vi "Day 14-Add to Pair Count.vi"(8 "Count":u64, 9 "Pair 2":u8[](array[numeric]), 10 "Pair 1":u8[](array[numeric]), 11 "Count in":map{u8[], u64}(c390)) -> (3 "Count out":map{u8[], u64}(c390))   [LabVIEW 2021]
uses:
  <vilib>/Utility/miscctls.llb/LVMapReplaceAction.ctl
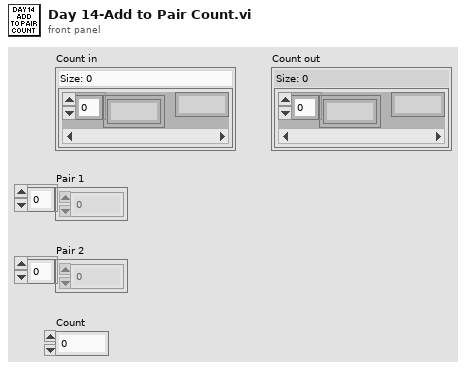
[diagram p1: front panel]
types:
  T1 = typedef "LVMapReplaceAction.ctl" = enum32{"Modify Entry only if found", "Add or Modify Entry", "Delete Entry"}
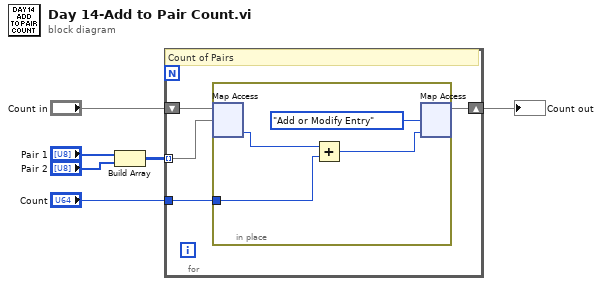
[diagram p0: block diagram]
diagram:
  n1 = Build Array("Pair 1", "Pair 2") -> (w1:u8[][])
  n2 = for {
    tunnel: w1 -> [w7] mode=indexing
    shift-right: [w8] -> w3
    shift-left: "Count in" -> [w9]
    tunnel: "Count" -> [w10]
    # "Count of Pairs"
    n3 = in-place {
      in-place-border: w10 -> [w11]
      n4 = in-place-map #1(w9, w7) -> (w13:u64)  [unwired: 1 in, 1 out]
      n5 = Add(x=w13, y=w11) -> (x+y=w12:u64)
      n6 = in-place-map #1(w12, LVMapReplaceAction."Add or Modify Entry" ("action")) -> (w8:map{u8[], u64})  [unwired: 2 out]
    }
  }
  "Count out" <- w3
